vi "IECMemory.Start.vi"(0 "i ref in":refnum<vi>, 2 "Ramp (F)":bool, 3 "ms timeout (100)":i32=100, 5 "error in (no error)":errorcluster) -> (14 "i ref out":refnum<vi>, 17 "timed out":bool, 19 "error out":errorcluster)   [LabVIEW 2014, in "IECMemory.lvlib"]
uses:
  IECMemory.lvlib
panel:
  # "NoRamp"
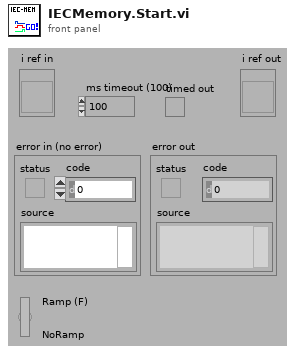
[diagram p1: front panel]
types:
  T1 = typedef "IECMemory.lvlib/IECMemory.i attribute.ctl" = cluster{"EndAddress":u32, "MemoryStatusBits":T2, "IEC Finished":bool, "Call Process":string, "Call Event":string}
  T2 = typedef "IECMemoryDriver.lvlib/Memory_Status.ctl" = bool[]
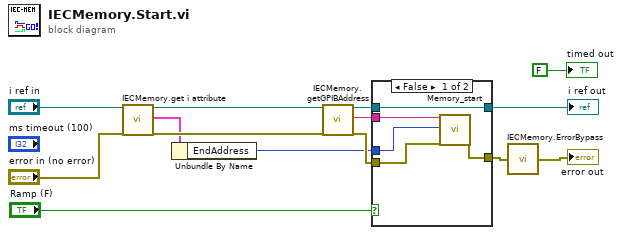
[diagram p0: block diagram]
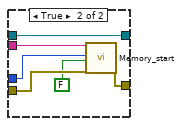
[diagram p2: hidden frame]
diagram:
  n1 = call "IECMemory.get i attribute.vi"("i ref in"="i ref in", "error in (no error)"="error in (no error)") -> ("i ref out"=w9:refnum<vi>, "i attribute"=w6:T1, "error out"=w8:errorcluster)  [unwired: 15 in]
  n2 = Unbundle By Name(w6) -> ("EndAddress"=w5:u32)
  n3 = call "IECMemory.getGPIBAddress.vi"("i ref in"=w9, "error in (no error)"=w8) -> ("i ref out"=w3:refnum<vi>, "GPIBAddress"=w14:string, "error out"=w13:errorcluster)  [unwired: 14 in, 1 out]
  n4 = case shown="False" "Ramp (F)" {
    tunnel: w14 -> [w19 w24]
    tunnel: w13 -> [w18 w22]
    tunnel: [w17 w23] -> w12
    tunnel: w5 -> [w16 w21]
    tunnel: [w15 w25] -> w2
    tunnel: w3 -> [w15 w25]
    frame False {
      n5 = call "Memory_start.vi"("address string"=w19, "EndAddress"=w16, "error in (no error)"=w18) -> ("error out"=w17:errorcluster)  [unwired: 16 in]
    }
    frame True {
      n6 = call "Memory_start.vi"("address string"=w24, "EndAddress"=w21, "TIMRAM (T)"=FALSE, "error in (no error)"=w22) -> ("error out"=w23:errorcluster)  [unwired: 15 in]
    }
  }
  "i ref out" <- w2
  n7 = call "IECMemory.ErrorBypass.vi"("error in (no error)"=w12) -> ("error out"=→"error out":errorcluster)  [unwired: 14 in]
  "timed out" <- FALSE ("timed out")
